vi "Credentials Dialog.vi"() -> (3 "Azure Credentials out":T1)   [LabVIEW 2015, in "_Unit Tests Shared.lvlib"]
uses:
  _Unit Tests Shared.lvlib
  Core/Azure Credentials.ctl
  Core/NI_Azure_Core.lvlib
panel:
  in  "OK":bool
  in  "Azure Credentials":T1
  # "Enter the Azure Credentials you wish to use for running these tests. Click OK when done."
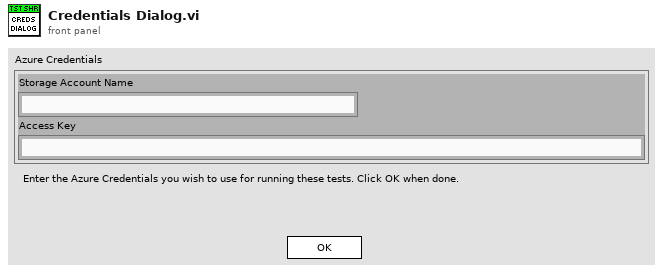
[diagram p1: front panel]
types:
  T1 = typedef "NI_Azure_Core.lvlib/Azure Credentials.ctl" = cluster{"Storage Account Name":string, "Access Key":string}
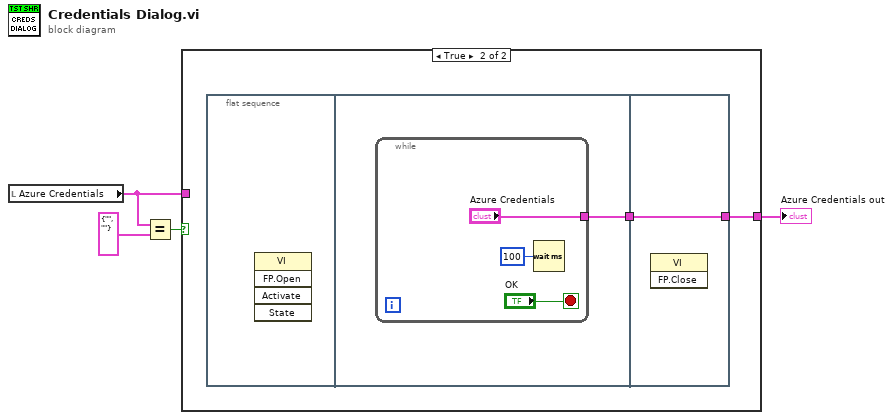
[diagram p0: block diagram]
diagram:
  n1 = local read "Azure Credentials"() -> (w1:T1)
  n2 = Equal?(x=w1, y=T1 {"Storage Account Name"="", "Access Key"=""}) -> (x = y?=w3:bool)
  n3 = case shown="True" w3 {
    tunnel: [w5 w7] -> w2
    tunnel: w1 -> [w5 _]
    frame False {
    }
    frame True {
      n4 = flat-sequence {
        tunnel: [w8] -> w6
        tunnel: [w12] -> w7
        tunnel: w6 -> [w12]
        frame #0 {
          n5 = invoke class="VI" method="FP.Open"() -> ()  [unwired: 5 in, 5 out]
        }
        frame #1 {
          n6 = while {
            tunnel: ["Azure Credentials"] -> w8
            stop <- "OK" stop-if-true
            n7 = Wait (ms)(milliseconds to wait=u32 100) -> ()  [unwired: 1 out]
          }
        }
        frame #2 {
          n8 = invoke class="VI" method="FP.Close"() -> ()  [unwired: 3 in, 3 out]
        }
      }
    }
  }
  "Azure Credentials out" <- w2
